vi "Host - ECAT Compatible Firmware.vi"(8 "error in (no error)":errorcluster, 11 "Slave Ref in":refnum<k21>) -> (0 "error out":errorcluster, 3 "Slave Ref out":refnum<k21>)   [LabVIEW 2019, in "SEECD System Explorer.lvlib"]
uses:
  SEECD System Explorer.lvlib
  <resource>/objmgr/IndComECAT.rc
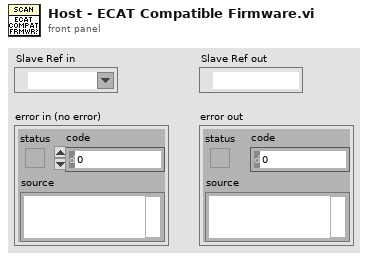
[diagram p1: front panel]
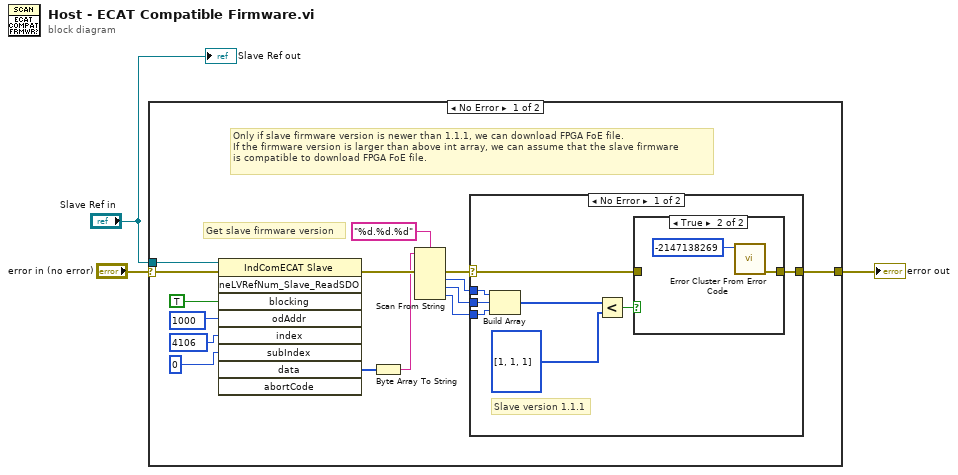
[diagram p0: block diagram]
diagram:
  n1 = case shown="No Error" "error in (no error)" {
    selector: "error in (no error)" -> [w4 w31]
    tunnel: [w18 w31] -> w3
    tunnel: "Slave Ref in" -> [w5 _]
    frame No Error {
      # "Only if slave firmware version is newer than 1.1.1, we can download FPGA FoE file.\nIf the firmware version is larger than above int array, we can assume that the slave firmware\nis compatible to download FPGA FoE file."
      # "Get slave firmware version"
      n2 = invoke class="IndComECAT Slave" method="neLVRefNum_Slave_ReadSDO"(reference=w5, error in=w4, "blocking"=TRUE, "odAddr"=u16 1000 ("odIndex"), "index"=u16 4106 ("odIndex"), "subIndex"=u8 0 ("SubIndex")) -> (error out=w12:errorcluster, "data"=w9:u8[])  [unwired: 3 in, 7 out]
      n3 = Byte Array To String(unsigned byte array=w9) -> (string=w11:string)
      n4 = Scan From String(format string="%d.%d.%d", input string=w11, error in=w12) -> (error out=w13:errorcluster, output 1=w14:i32, output 2=w15:i32, output 3=w16:i32)  [unwired: 4 in, 2 out]
      n5 = case shown="No Error" w13 {
        selector: w13 -> [w19 w30]
        tunnel: w14 -> [w26 _]
        tunnel: w15 -> [w25 _]
        tunnel: w16 -> [w24 _]
        tunnel: [w21 w30] -> w18
        frame No Error {
          # "Slave version 1.1.1"
          n6 = Build Array(w26, w25, w24) -> (w23:i32[])
          n7 = Less?(x=w23, y=i32[] [1, 1, 1]) -> (x < y?=w20:bool)
          n8 = case shown="True" w20 {
            tunnel: w19 -> [w27 _]
            tunnel: [w27 w28] -> w21
            frame False {
            }
            frame True {
              n9 = call <vilib>:"Error Cluster From Error Code.vi"("error code (0)"=-2147138269) -> ("error out"=w28:errorcluster)  [unwired: 8 in]
            }
          }
        }
        frame Error {
        }
      }
    }
    frame Error {
    }
  }
  "error out" <- w3
  "Slave Ref out" <- "Slave Ref in"
